vi "String Insert Tests.vi"() -> ()   [LabVIEW 2021]
uses:
  <vilib>/numeric/Random Number (Range) U64.vi
  <vilib>/numeric/sub_Random U32.vi
panel:
  out "x-y":dbl
  out "Result":string
  in  "Offset":i32
  in  "Insert":string
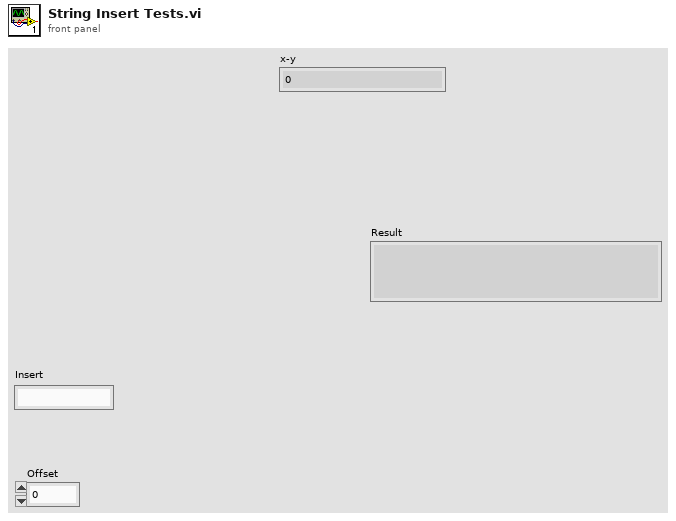
[diagram p1: front panel]
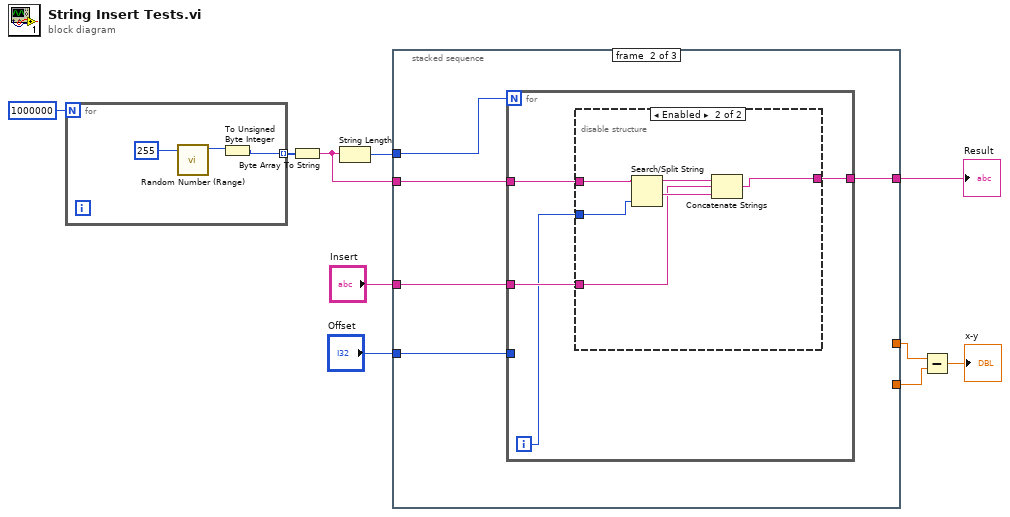
[diagram p0: block diagram]
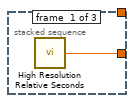
[diagram p2: hidden frame]
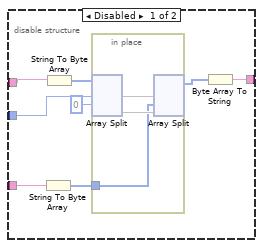
[diagram p3: hidden frame]
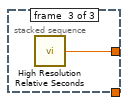
[diagram p4: hidden frame]
diagram:
  n1 = for {
    N: 1000000 -> [_]
    tunnel: [w11] -> w2 mode=indexing
    n2 = call-poly <vilib>:"Random Number (Range).vi"("upper bound (100)"=u64 255) -> ("number"=w12:u64)  [unwired: 10 in]
    n3 = To Unsigned Byte Integer(number=w12) -> (unsigned 8bit integer=w11:u8)
  }
  n4 = Byte Array To String(unsigned byte array=w2) -> (string=w1:string)
  n5 = String Length(string=w1) -> (length=w4:i32)
  n6 = stacked-sequence {
    tunnel: w1 -> [_ w16 _]
    tunnel: "Insert" -> [_ w19 _]
    tunnel: "Offset" -> [_ w18 _]
    tunnel: [_ w15 _] -> w8
    tunnel: [w14 _ _] -> w6
    tunnel: [_ _ w41] -> w7
    tunnel: w4 -> [_ w17 _]
    frame #0 {
      n7 = call <vilib>:"High Resolution Relative Seconds.vi"() -> ("relative seconds"=w14:dbl)
    }
    frame #1 {
      n8 = for {
        N: w17 -> [_]
        tunnel: w16 -> [w21]
        tunnel: w19 -> [w23]
        tunnel: w18 -> [_]
        tunnel: [w20] -> w15
        i -> [w22]
        n9 = disable-structure shown="Enabled" {
          disable-tunnel: w23 -> [w31 w36]
          disable-tunnel: w22 -> [w30 w39]
          disable-tunnel: w21 -> [w29 w40]
          disable-tunnel: [w28 w35] -> w20
          frame Disabled {
            n10 = String To Byte Array(string=w31) -> (unsigned byte array=w27:u8[])
            n11 = String To Byte Array(string=w29) -> (unsigned byte array=w26:u8[])
            n12 = in-place {
              in-place-border: w27 -> [w32]
              n13 = in-place-split #1(w26, w30, 0) -> (w34:u8[], w33:u8[])  [unwired: 1 out]
              n14 = in-place-split #1(w34, w32, w33) -> (w24:u8[])  [unwired: 2 out]
            }
            n15 = Byte Array To String(unsigned byte array=w24) -> (string=w28:string)
          }
          frame Enabled {
            n16 = Search/Split String(string=w40, offset (0)=w39) -> (substring before match=w38:string, match + rest of string=w37:string)  [unwired: 1 in, 1 out]
            n17 = Concatenate Strings(w38, w36, w37) -> (w35:string)
          }
        }
      }
    }
    frame #2 {
      n18 = call <vilib>:"High Resolution Relative Seconds.vi"() -> ("relative seconds"=w41:dbl)
    }
  }
  "Result" <- w8
  n19 = Subtract(x=w7, y=w6) -> (x-y=→"x-y":dbl)
